vi "oax_Generate Piecewise Signal (block).vi"(4 "acc transition ratio":dbl=0.1, 6 "order":dbl, 7 "fs":dbl, 8 "init phase":dbl, 9 "passed samples in":cluster{"pre":dbl, "mid":dbl, "post":dbl}, 11 "position":T1) -> (0 "final phase":dbl, 1 "passed samples out":cluster{"pre":dbl, "mid":dbl, "post":dbl}, 3 "phase out":dbl[](array[numeric]))   [LabVIEW 2017]
uses:
  <vilib>/Analysis/1siggen.llb/Ramp Pattern by Samples.vi
  <vilib>/Analysis/NI_AALBase.lvlib
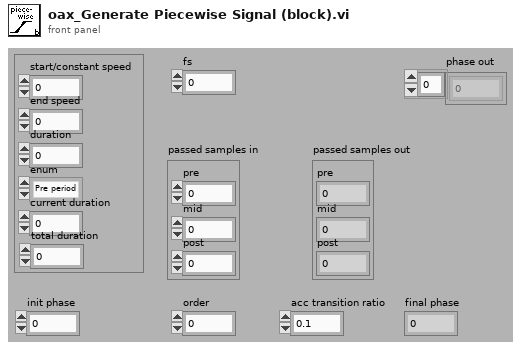
[diagram p1: front panel]
types:
  T1 = cluster{"start/constant speed":dbl, "end speed":dbl, "duration":dbl, "enum":enum16{"Pre period", "Middle period", "Post period"}, "current duration":dbl, "total duration":dbl}
  T2 = enum16{"Pre period", "Middle period", "Post period"}
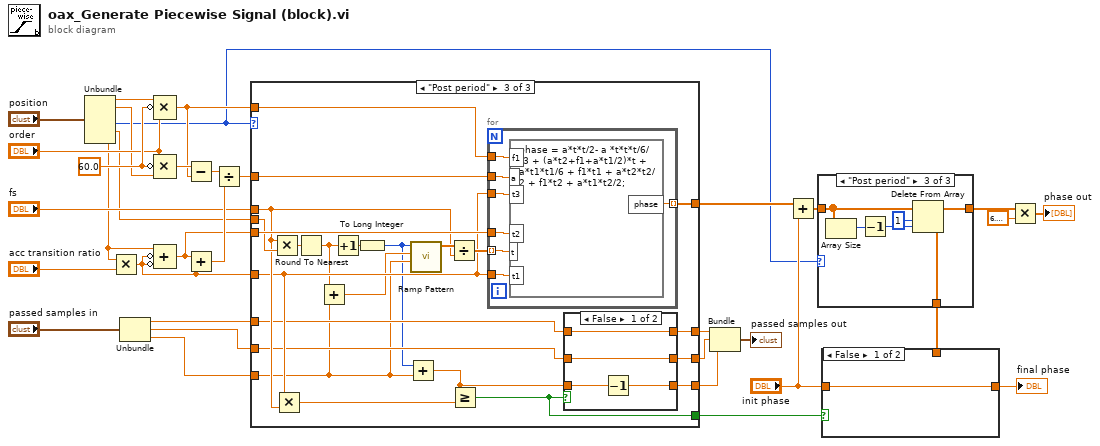
[diagram p0: block diagram]
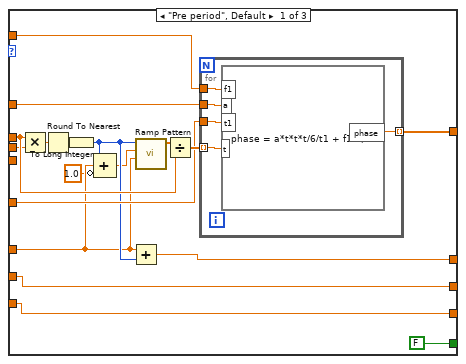
[diagram p2: hidden frame]
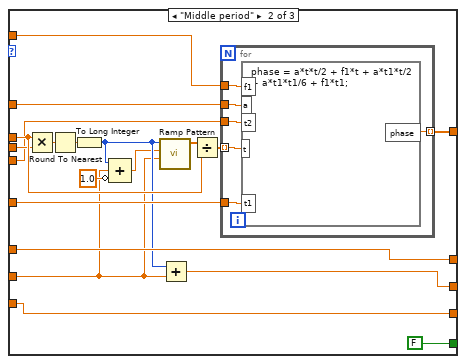
[diagram p3: hidden frame]
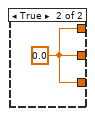
[diagram p4: hidden frame]
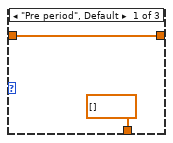
[diagram p5: hidden frame]
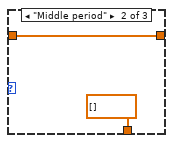
[diagram p6: hidden frame]
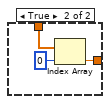
[diagram p7: hidden frame]
diagram:
  w33 = 60.0 ("y")
  n1 = Unbundle("position") -> ("start/constant speed"=w25:dbl, "end speed"=w24:dbl, "enum"=w9:T2, "current duration"=w19:dbl, "total duration"=w18:dbl)  [unwired: 1 out]
  n2 = Multiply(x=w18, y="acc transition ratio") -> (x*y=w15:dbl)
  n3 = Unbundle("passed samples in") -> ("pre"=w7:dbl, "mid"=w6:dbl, "post"=w5:dbl)
  n4 = Compound Arithmetic op=MULTIPLY(w25, invert w33, "order") -> (w22:dbl)
  n5 = Compound Arithmetic op=MULTIPLY("order", invert w33, w24) -> (w31:dbl)
  n6 = Compound Arithmetic op=ADD(w18, invert w15, invert w15) -> (w16:dbl)
  n7 = Subtract(x=w31, y=w22) -> (x-y=w29:dbl)
  n8 = Add(x=w16, y=w15) -> (x+y=w28:dbl)
  n9 = Divide(x=w29, y=w28) -> (x/y=w23:dbl)
  n10 = case shown="\"Post period\"" w9 {
    tunnel: "fs" -> [w50 w68 w96]
    tunnel: w19 -> [w46 w63 w98]
    tunnel: w23 -> [w47 w71 w103]
    tunnel: w22 -> [w45 w70 w101]
    tunnel: [w49 w72 w102] -> w20
    tunnel: w15 -> [w39 w69 w95]
    tunnel: w16 -> [_ w62 w100]
    tunnel: [FALSE FALSE w94] -> w11
    tunnel: [w40 w66 w93] -> w4
    tunnel: w7 -> [w37 w66 w90]
    tunnel: [w42 w64 w92] -> w3
    tunnel: w6 -> [w42 w59 w89]
    tunnel: [w41 w65 w91] -> w2
    tunnel: w5 -> [w41 w65 w85]
    frame "Pre period", Default {
      n11 = Multiply(x=w50, y=w46) -> (x*y=w51:dbl)
      n12 = Round To Nearest(number=w51) -> (nearest integer value=w44:dbl)
      n13 = To Long Integer(number=w44) -> (32bit integer=w38:i32)
      n14 = Compound Arithmetic op=ADD(w38, w37, invert 1.0 ("value")) -> (w35:dbl)
      n15 = Add(x=w37, y=w38) -> (x+y=w40:dbl)
      n16 = call-poly <vilib>:"Ramp Pattern.vi"("start"=w37, "end"=w35, "samples"=w38) -> ("Ramp Pattern"=w52:dbl[])  [unwired: 7 in, 1 out]
      n17 = Divide(x=w52, y=w50) -> (x/y=w48:dbl[])
      n18 = for {
        tunnel: w47 -> [w57]
        tunnel: w39 -> [w56]
        tunnel: w45 -> [w55]
        tunnel: w48 -> [w54] mode=indexing
        tunnel: [w53] -> w49 mode=indexing
        n19 = formula code="phase = a*t*t*t/6/t1 + f1*t;"("a"=w57, "t"=w54, "t1"=w56, "f1"=w55) -> ("phase"=w53:dbl)
      }
    }
    frame "Middle period" {
      n20 = Multiply(x=w68, y=w63) -> (x*y=w75:dbl)
      n21 = Round To Nearest(number=w75) -> (nearest integer value=w73:dbl)
      n22 = To Long Integer(number=w73) -> (32bit integer=w60:i32)
      n23 = Compound Arithmetic op=ADD(w60, w59, invert 1.0 ("value")) -> (w58:dbl)
      n24 = call-poly <vilib>:"Ramp Pattern.vi"("start"=w59, "end"=w58, "samples"=w60) -> ("Ramp Pattern"=w76:dbl[])  [unwired: 7 in, 1 out]
      n25 = Add(x=w60, y=w59) -> (x+y=w64:dbl)
      n26 = Divide(x=w76, y=w68) -> (x/y=w74:dbl[])
      n27 = for {
        tunnel: w71 -> [w82]
        tunnel: w69 -> [w81]
        tunnel: w62 -> [w80]
        tunnel: w70 -> [w79]
        tunnel: w74 -> [w78] mode=indexing
        tunnel: [w77] -> w72 mode=indexing
        n28 = formula code="phase = a*t*t/2 + f1*t + a*t1*t/2 + a*t1*t1/6 + f1*t1;"("a"=w82, "t"=w78, "t1"=w81, "t2"=w80, "f1"=w79) -> ("phase"=w77:dbl)
      }
    }
    frame "Post period" {
      n29 = Multiply(x=w96, y=w98) -> (x*y=w97:dbl)
      n30 = Multiply(x=w95, y=w96) -> (x*y=w99:dbl)
      n31 = Round To Nearest(number=w97) -> (nearest integer value=w86:dbl)
      n32 = Add(x=w86, y=w85) -> (x+y=w88:dbl)
      n33 = Increment(x=w86) -> (x+1=w87:dbl)
      n34 = To Long Integer(number=w87) -> (32bit integer=w84:i32)
      n35 = Add(x=w84, y=w85) -> (x+y=w83:dbl)
      n36 = call-poly <vilib>:"Ramp Pattern.vi"("start"=w85, "end"=w88, "samples"=w84) -> ("Ramp Pattern"=w105:dbl[])  [unwired: 7 in, 1 out]
      n37 = Divide(x=w105, y=w96) -> (x/y=w104:dbl[])
      n38 = Greater Or Equal?(x=w83, y=w99) -> (x >= y?=w94:bool)
      n39 = for {
        tunnel: w103 -> [w117]
        tunnel: w95 -> [w116]
        tunnel: w100 -> [w115]
        tunnel: w95 -> [w114]
        tunnel: w101 -> [w113]
        tunnel: w104 -> [w112] mode=indexing
        tunnel: [w111] -> w102 mode=indexing
        n40 = formula code="phase = a*t*t/2- a *t*t*t/6/t3 + (a*t2+f1+a*t1/2)*t + a*t1*t1/6 + f1*t1 + a*t2*t2/2 + f1*t2 + a*t1*t2/2;"("a"=w117, "t"=w112, "t1"=w116, "t2"=w115, "t3"=w114, "f1"=w113) -> ("phase"=w111:dbl)
      }
      n41 = case shown="False" w94 {
        tunnel: [w109 w110] -> w93
        tunnel: [w108 w110] -> w92
        tunnel: [w106 w110] -> w91
        tunnel: w90 -> [w109 _]
        tunnel: w89 -> [w108 _]
        tunnel: w83 -> [w107 _]
        frame False {
          n42 = Decrement(x=w107) -> (x-1=w106:dbl)
        }
        frame True {
          w110 = 0.0
        }
      }
    }
  }
  n43 = Bundle("pre"=w4, "mid"=w3, "post"=w2) -> (→"passed samples out":cluster{"pre":dbl, "mid":dbl, "post":dbl})  [unwired: 1 in]
  n44 = Add(x=w20, y="init phase") -> (x+y=w17:dbl[])
  n45 = case shown="\"Post period\"" w9 {
    tunnel: w17 -> [w119 w121 w127]
    tunnel: [dbl[] [] dbl[] [] w125] -> w13
    tunnel: [w119 w121 w122] -> w12
    frame "Pre period", Default {
    }
    frame "Middle period" {
    }
    frame "Post period" {
      n46 = Array Size(array=w127) -> (size(s)=w124:i32)
      n47 = Decrement(x=w124) -> (x-1=w123:i32)
      n48 = Delete From Array(array=w127, length=1, index=w123) -> (deleted portion=w125:dbl[], array with subset deleted=w122:dbl[])
    }
  }
  n49 = case shown="False" w11 {
    tunnel: [w128 w131] -> w27
    tunnel: w13 -> [_ w130]
    tunnel: "init phase" -> [w128 _]
    frame False {
    }
    frame True {
      n50 = Index Array(array=w130, index=0) -> (element=w131:dbl)
    }
  }
  "final phase" <- w27
  n51 = Multiply(x=w12, y=6.283185307179586) -> (x*y=→"phase out":dbl[])
